vi "DVR - Initialize DVRs.vi"(8 "error in":errorcluster, 11 "EMS Generic in":refnum<class "EMS Generic.lvclass">) -> (0 "error out":errorcluster, 3 "EMS Generic out":refnum<class "EMS Generic.lvclass">)   [LabVIEW 2018, in "EMS Generic Actor.lvlib" / "EMS Generic.lvclass"]
uses:
  EMS Generic.lvclass
  Controls/Data Type DVRs.ctl
  EMS Generic.lvclass/EMS Generic.ctl
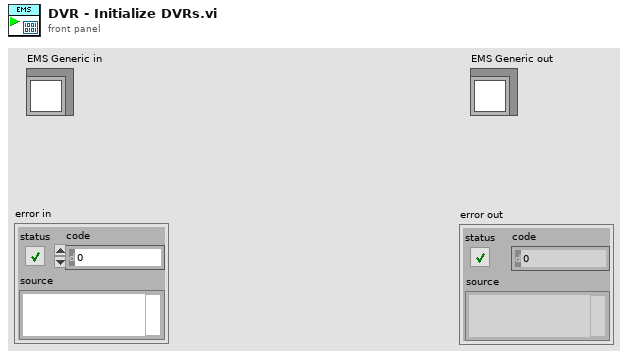
[diagram p1: front panel]
types:
  T1 = typedef "EMS Generic Actor.lvlib/EMS Generic.lvclass/Data Type DVRs.ctl" = cluster{"IED_Status":refnum<data-value>, "IED_Status_0":refnum<data-value>, "DER_Measurement":refnum<data-value>, "DER_Info":refnum<data-value>, "DER_Status":refnum<data-value>, "ES_Measurement":refnum<data-value>, "ES_Info":refnum<data-value>, "PV_Info":refnum<data-value>, "SmartRelay_Info":refnum<data-value>, "SmartRelay_Measurement":refnum<data-value>, "Meter_Info":refnum<data-value>, "Meter_Measurement":refnum<data-value>, "HVAC_Status":refnum<data-value>, "HVAC_Measurement":refnum<data-value>, "PriceData_RealTime":refnum<data-value>, "PriceData_Demand":refnum<data-value>, "PriceData_Energy":refnum<data-value>, "ForecastData_Long":refnum<data-value>, "ForecastData_Short":refnum<data-value>, "DER_Control":refnum<data-value>, "DER_SetPointF":refnum<data-value>, "DER_SetPointP":refnum<data-value>, "DER_SetPointQ":refnum<data-value>, "DER_SetPointPF":refnum<data-value>, "DER_SetPointV":refnum<data-value>, "PV_setCurtailment":refnum<data-value>, "PV_setRampRate":refnum<data-value>, "Relay_Control":refnum<data-value>, "Load_Control":refnum<data-value>, "HVAC_Control":refnum<data-value>, "Generator_Info":refnum<data-value>, "ForecastData_Long_Backup":refnum<data-value>, "PriceData_RealTime_Backup":refnum<data-value>}
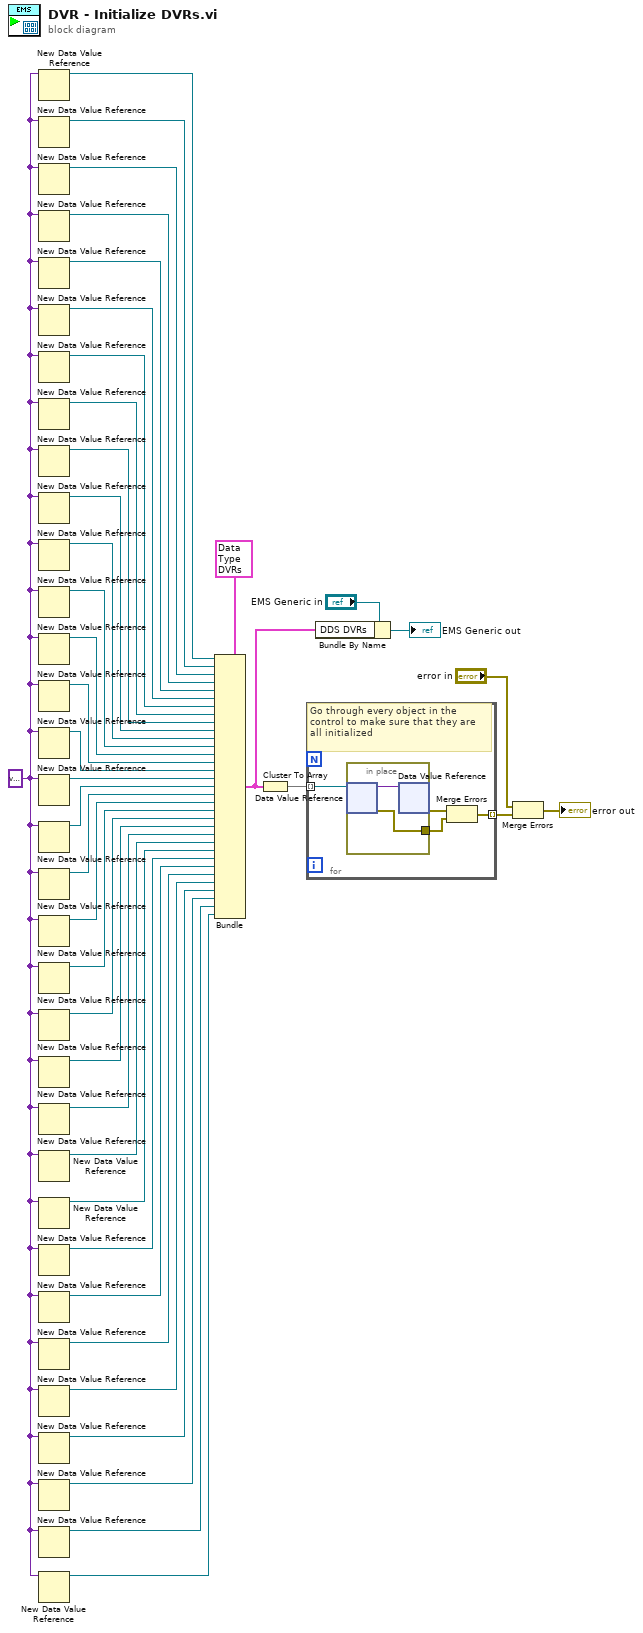
[diagram p0: block diagram]
diagram:
  w2 = variant
  n1 = New Data Value Reference(data value=w2) -> (data value reference=w29:refnum<data-value>)  [unwired: 1 in, 1 out]
  n2 = New Data Value Reference(data value=w2) -> (data value reference=w24:refnum<data-value>)  [unwired: 1 in, 1 out]
  n3 = New Data Value Reference(data value=w2) -> (data value reference=w25:refnum<data-value>)  [unwired: 1 in, 1 out]
  n4 = New Data Value Reference(data value=w2) -> (data value reference=w26:refnum<data-value>)  [unwired: 1 in, 1 out]
  n5 = New Data Value Reference(data value=w2) -> (data value reference=w27:refnum<data-value>)  [unwired: 1 in, 1 out]
  n6 = New Data Value Reference(data value=w2) -> (data value reference=w28:refnum<data-value>)  [unwired: 1 in, 1 out]
  n7 = New Data Value Reference(data value=w2) -> (data value reference=w30:refnum<data-value>)  [unwired: 1 in, 1 out]
  n8 = New Data Value Reference(data value=w2) -> (data value reference=w31:refnum<data-value>)  [unwired: 1 in, 1 out]
  n9 = New Data Value Reference(data value=w2) -> (data value reference=w32:refnum<data-value>)  [unwired: 1 in, 1 out]
  n10 = New Data Value Reference(data value=w2) -> (data value reference=w33:refnum<data-value>)  [unwired: 1 in, 1 out]
  n11 = New Data Value Reference(data value=w2) -> (data value reference=w34:refnum<data-value>)  [unwired: 1 in, 1 out]
  n12 = New Data Value Reference(data value=w2) -> (data value reference=w35:refnum<data-value>)  [unwired: 1 in, 1 out]
  n13 = New Data Value Reference(data value=w2) -> (data value reference=w36:refnum<data-value>)  [unwired: 1 in, 1 out]
  n14 = New Data Value Reference(data value=w2) -> (data value reference=w37:refnum<data-value>)  [unwired: 1 in, 1 out]
  n15 = New Data Value Reference(data value=w2) -> (data value reference=w38:refnum<data-value>)  [unwired: 1 in, 1 out]
  n16 = New Data Value Reference(data value=w2) -> (data value reference=w40:refnum<data-value>)  [unwired: 1 in, 1 out]
  n17 = New Data Value Reference(data value=w2) -> (data value reference=w23:refnum<data-value>)  [unwired: 1 in, 1 out]
  n18 = New Data Value Reference(data value=w2) -> (data value reference=w22:refnum<data-value>)  [unwired: 1 in, 1 out]
  n19 = New Data Value Reference(data value=w2) -> (data value reference=w21:refnum<data-value>)  [unwired: 1 in, 1 out]
  n20 = New Data Value Reference(data value=w2) -> (data value reference=w20:refnum<data-value>)  [unwired: 1 in, 1 out]
  n21 = New Data Value Reference(data value=w2) -> (data value reference=w19:refnum<data-value>)  [unwired: 1 in, 1 out]
  n22 = New Data Value Reference(data value=w2) -> (data value reference=w18:refnum<data-value>)  [unwired: 1 in, 1 out]
  n23 = New Data Value Reference(data value=w2) -> (data value reference=w17:refnum<data-value>)  [unwired: 1 in, 1 out]
  n24 = New Data Value Reference(data value=w2) -> (data value reference=w16:refnum<data-value>)  [unwired: 1 in, 1 out]
  n25 = New Data Value Reference(data value=w2) -> (data value reference=w15:refnum<data-value>)  [unwired: 1 in, 1 out]
  n26 = New Data Value Reference(data value=w2) -> (data value reference=w14:refnum<data-value>)  [unwired: 1 in, 1 out]
  n27 = New Data Value Reference(data value=w2) -> (data value reference=w13:refnum<data-value>)  [unwired: 1 in, 1 out]
  n28 = New Data Value Reference(data value=w2) -> (data value reference=w12:refnum<data-value>)  [unwired: 1 in, 1 out]
  n29 = New Data Value Reference(data value=w2) -> (data value reference=w11:refnum<data-value>)  [unwired: 1 in, 1 out]
  n30 = New Data Value Reference(data value=w2) -> (data value reference=w10:refnum<data-value>)  [unwired: 1 in, 1 out]
  n31 = New Data Value Reference(data value=w2) -> (data value reference=w9:refnum<data-value>)  [unwired: 1 in, 1 out]
  n32 = New Data Value Reference(data value=w2) -> (data value reference=w8:refnum<data-value>)  [unwired: 1 in, 1 out]
  n33 = New Data Value Reference(data value=w2) -> (data value reference=w1:refnum<data-value>)  [unwired: 1 in, 1 out]
  n34 = Bundle(cluster=T1 {"IED_Status"=refnum, "IED_Status_0"=refnum, "DER_Measurement"=refnum, "DER_Info"=refnum, "DER_Status"=refnum, "ES_Measurement"=refnum, "ES_Info"=refnum, "PV_Info"=refnum, "SmartRelay_Info"=refnum, "SmartRelay_Measurement"=refnum, "Meter_Info"=refnum, "Meter_Measurement"=refnum, "HVAC_Status"=refnum, "HVAC_Measurement"=refnum, "PriceData_RealTime"=refnum, "PriceData_Demand"=refnum, "PriceData_Energy"=refnum, "ForecastData_Long"=refnum, "ForecastData_Short"=refnum, "DER_Control"=refnum, "DER_SetPointF"=refnum, "DER_SetPointP"=refnum, "DER_SetPointQ"=refnum, "DER_SetPointPF"=refnum, "DER_SetPointV"=refnum, "PV_setCurtailment"=refnum, "PV_setRampRate"=refnum, "Relay_Control"=refnum, "Load_Control"=refnum, "HVAC_Control"=refnum, "Generator_Info"=refnum, "ForecastData_Long_Backup"=refnum, "PriceData_RealTime_Backup"=refnum} ("DVR"), "IED_Status"=w29, "IED_Status_0"=w24, "DER_Measurement"=w25, "DER_Info"=w26, "DER_Status"=w27, "ES_Measurement"=w28, "ES_Info"=w30, "PV_Info"=w31, "SmartRelay_Info"=w32, "SmartRelay_Measurement"=w33, "Meter_Info"=w34, "Meter_Measurement"=w35, "HVAC_Status"=w36, "HVAC_Measurement"=w37, "PriceData_RealTime"=w38, "PriceData_Demand"=w40, "PriceData_Energy"=w23, "ForecastData_Long"=w22, "ForecastData_Short"=w21, "DER_Control"=w20, "DER_SetPointF"=w19, "DER_SetPointP"=w18, "DER_SetPointQ"=w17, "DER_SetPointPF"=w16, "DER_SetPointV"=w15, "PV_setCurtailment"=w14, "PV_setRampRate"=w13, "Relay_Control"=w12, "Load_Control"=w11, "HVAC_Control"=w10, "Generator_Info"=w9, "ForecastData_Long_Backup"=w8, "PriceData_RealTime_Backup"=w1) -> (w5:T1)
  n35 = Cluster To Array(cluster=w5) -> (array=w6:refnum<data-value>[])
  n36 = for {
    tunnel: w6 -> [w46] mode=indexing
    tunnel: [w44] -> w7 mode=indexing
    # "Go through every object in the control to make sure that they are all initialized"
    n37 = in-place {
      in-place-border: [w47] -> w45
      n38 = in-place-dvr #1(w46) -> (w48:variant, w47:errorcluster)
      n39 = in-place-dvr #1(w48) -> (w43:errorcluster)  [unwired: 1 out]
    }
    n40 = Merge Errors(w43, w45) -> (w44:errorcluster)
  }
  n41 = Bundle By Name(cluster="EMS Generic in", "DDS DVRs"=w5) -> (→"EMS Generic out":refnum<class "EMS Generic.lvclass">)
  n42 = Merge Errors("error in", w7) -> (→"error out":errorcluster)
